vi "Read ControlStatus.vi"(8 "error in (no error)":errorcluster, 11 "CoolerControler in":refnum<class "CoolerControler.lvclass">) -> (0 "error out":errorcluster, 2 "Status":T1, 3 "CoolerControler out":refnum<class "CoolerControler.lvclass">)   [LabVIEW 2016, in "CoolerControler.lvclass"]
uses:
  CoolerControler.lvclass
  typedefs/DeviceStatus.ctl
  typedefs/ControlStatusMode.ctl
  typedefs/PumpStatusFlag.ctl
  typedefs/AlarmStatusFlag.ctl
  typedefs/WarningStatusFlag.ctl
  CoolerControler.lvclass/CoolerControler.ctl
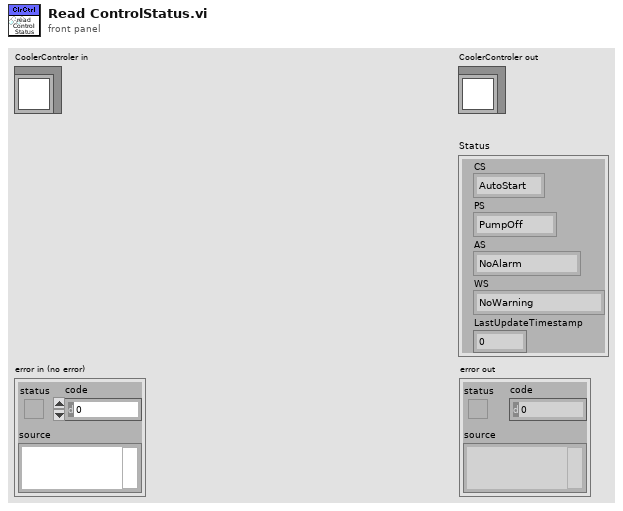
[diagram p1: front panel]
types:
  T1 = typedef "DeviceStatus.ctl" = cluster{"CS":T2, "PS":T3, "AS":T4, "WS":T5, "LastUpdateTimestamp":dbl}
  T2 = typedef "ControlStatusMode.ctl" = enum16{"AutoStart", "Standby", "Run", "Safety", "Test"}
  T3 = typedef "PumpStatusFlag.ctl" = enum16{"PumpOff", "PumpOn"}
  T4 = typedef "AlarmStatusFlag.ctl" = enum16{"NoAlarm", "AlarmPresent"}
  T5 = typedef "WarningStatusFlag.ctl" = enum16{"NoWarning", "WarningPresent"}
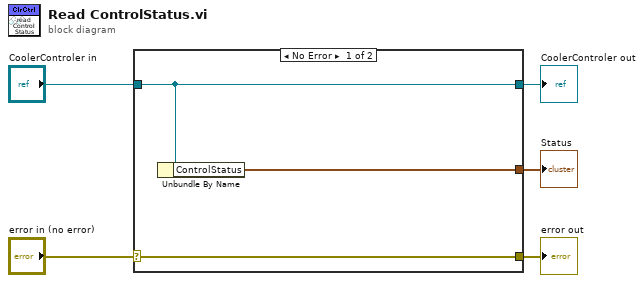
[diagram p0: block diagram]
diagram:
  n1 = case shown="No Error" "error in (no error)" {
    selector: "error in (no error)" -> [w8 w9]
    tunnel: [w8 w9] -> w4
    tunnel: [w7 w10] -> w2
    tunnel: "CoolerControler in" -> [w7 w10]
    tunnel: [w6 _] -> w1
    frame No Error {
      n2 = Unbundle By Name(w7) -> ("ControlStatus"=w6:T1)
    }
    frame Error {
    }
  }
  "error out" <- w4
  "CoolerControler out" <- w2
  "Status" <- w1
